vi "MSG New Data For GUI.vi"(8 "error in":errorcluster, 10 "data":variant) -> (0 "error out":errorcluster)   [LabVIEW 2020, in "Manager.lvlib"]
doc: "Send component-specific API message: ERROR"
uses:
  Manager.lvlib
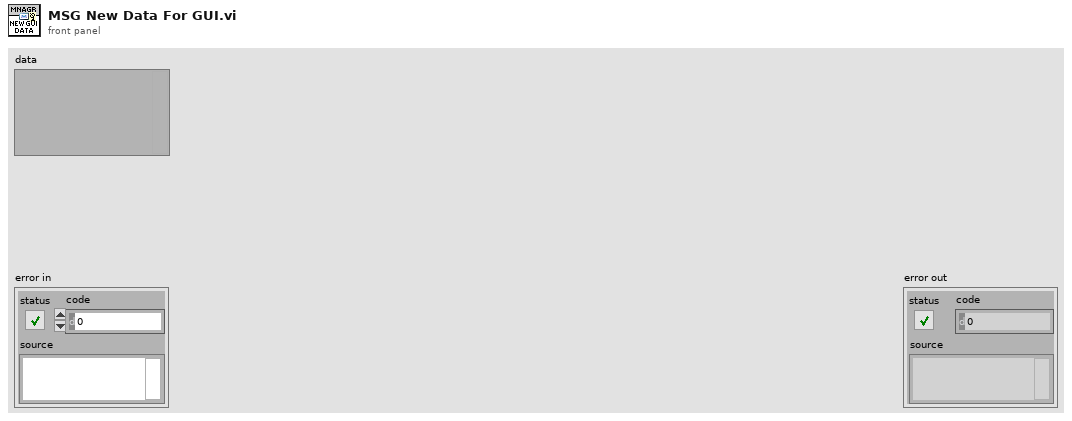
[diagram p1: front panel]
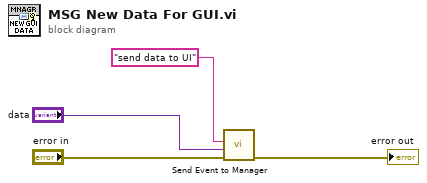
[diagram p0: block diagram]
diagram:
  n1 = call "Send Event to Manager.vi"("error in"="error in", "Payload"="data", "Command"="send data to UI") -> ("error out"=→"error out":errorcluster)  [unwired: 8 in]
